vi "SSH_TUNNEL_ResetOpenConnections.vi"(8 "error in (no error)":errorcluster, 11 "SSH_TUNNEL in":refnum<class "SSH_TUNNEL.lvclass">) -> (0 "error out":errorcluster, 3 "SSH_TUNNEL out":refnum<class "SSH_TUNNEL.lvclass">)   [LabVIEW 2018, in "SSH_TUNNEL.lvclass"]
uses:
  SSH_TUNNEL.lvclass
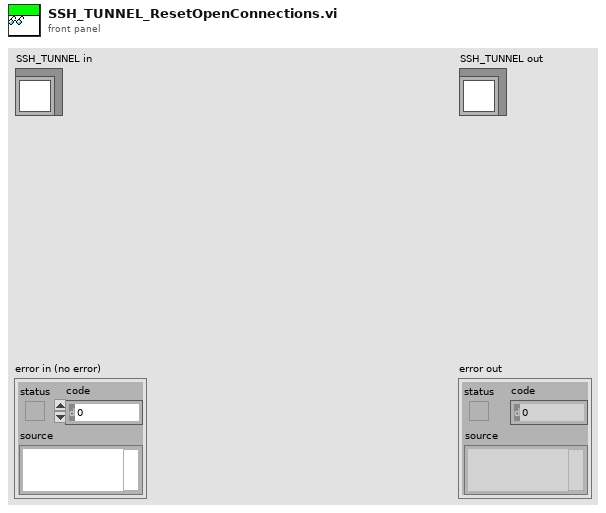
[diagram p1: front panel]
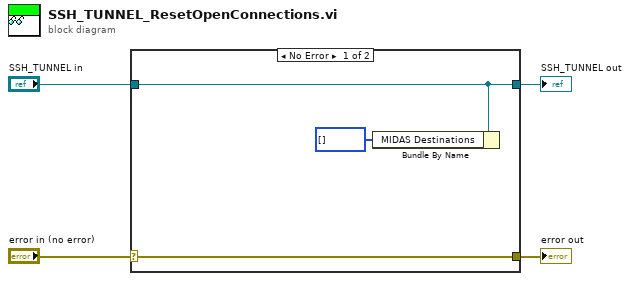
[diagram p0: block diagram]
diagram:
  n1 = case shown="No Error" "error in (no error)" {
    selector: "error in (no error)" -> [w7 w8]
    tunnel: [w7 w8] -> w3
    tunnel: [w6 w9] -> w1
    tunnel: "SSH_TUNNEL in" -> [w6 w9]
    frame No Error {
      n2 = Bundle By Name(cluster=w6, "MIDAS Destinations"=u16[] [] ("Open Connections")) -> ()  [unwired: 1 out]
    }
    frame Error {
    }
  }
  "error out" <- w3
  "SSH_TUNNEL out" <- w1
